vi "短信服务全局变量.vi"() -> ()   [LabVIEW 2016, in "Alarm interface.lvlib" / "短信语音库.lvlib"]
panel:
  in  "PN3":T1
  in  "PN2":T1
  in  "PN1":T1
  in  "启用":bool
  in  "站点":string
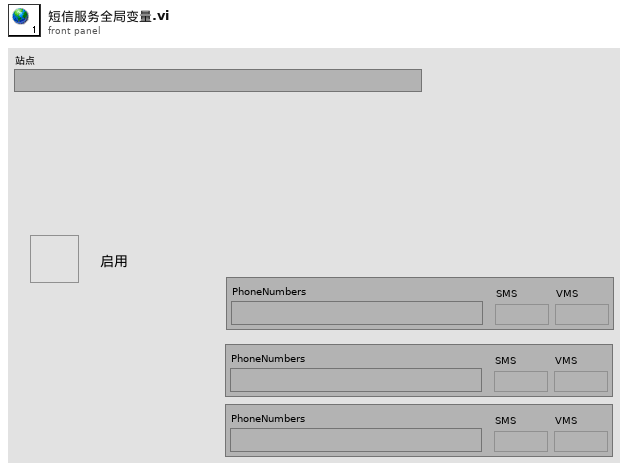
[diagram p1: front panel]
types:
  T1 = cluster{"PhoneNumbers":string, "SMS":bool, "VMS":bool}
diagram:
